vi "Configure Waveform Setup.vi"(4 "Number of points (0: All points)":i16, 6 "Segment number (0: All segment)":i16, 7 "First point (0: First point)":i16, 8 "error in (no error)":errorcluster, 9 "Sparsing (0: Every point)":i16, 11 "VISA resource name":refnum<visa-resource-name>) -> (0 "error out":errorcluster, 3 "VISA resource name out":refnum<visa-resource-name>)   [LabVIEW 2020, in "LeCroy Wave Series.lvlib"]
doc: "The waveform setup command specifies the amount of data in a waveform to be transmitted to the controller."
uses:
  LeCroy Wave Series.lvlib
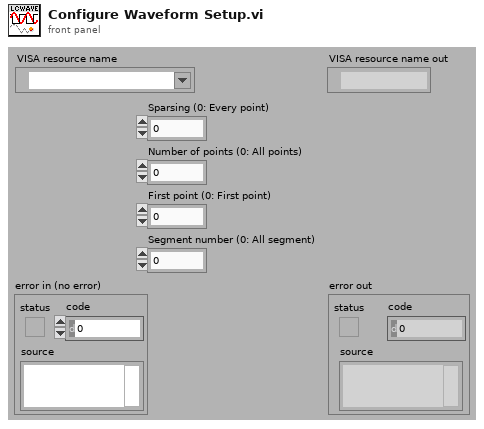
[diagram p1: front panel]
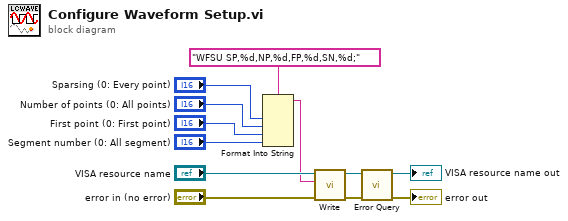
[diagram p0: block diagram]
diagram:
  n1 = Format Into String(format string="WFSU SP,%d,NP,%d,FP,%d,SN,%d;", "Sparsing (0: Every point)", "Number of points (0: All points)", "First point (0: First point)", "Segment number (0: All segment)") -> (resulting string=w5:string)  [unwired: 2 in, 1 out]
  n2 = call "Write.vi"("error in (no error)"="error in (no error)", "Write Buffer"=w5, "VISA resource name"="VISA resource name") -> ("error out"=w3:errorcluster, "VISA resource name out"=w4:refnum<visa-resource-name>)  [unwired: 6 in, 1 out]
  n3 = call "Error Query.vi"("error in (no error)"=w3, "VISA resource name"=w4) -> ("error out"=→"error out":errorcluster, "VISA resource name out"=→"VISA resource name out":refnum<visa-resource-name>)  [unwired: 6 in, 2 out]
